vi "Main.vi"() -> ()   [LabVIEW 2024]
uses:
  PIMax3Test01/x64/Debug/PIMax3Test02.dll
panel:
  in  "Accumulations":i64
  out "Accumulations (Get)":i64
  out "Close Camera":string
  out "Intensity Graph 2":u16[][](graph)
  out "Uninit Message":string
  out "model":string
  out "open":string
  out "Init Message":string
  out "Uninit Code":i32
  out "Init Code":i32
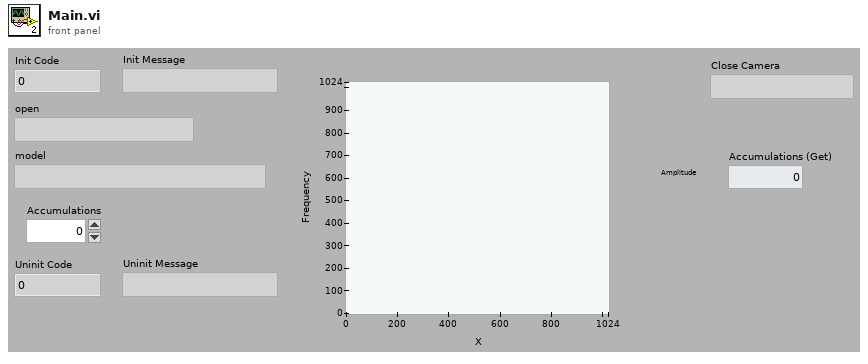
[diagram p1: front panel]
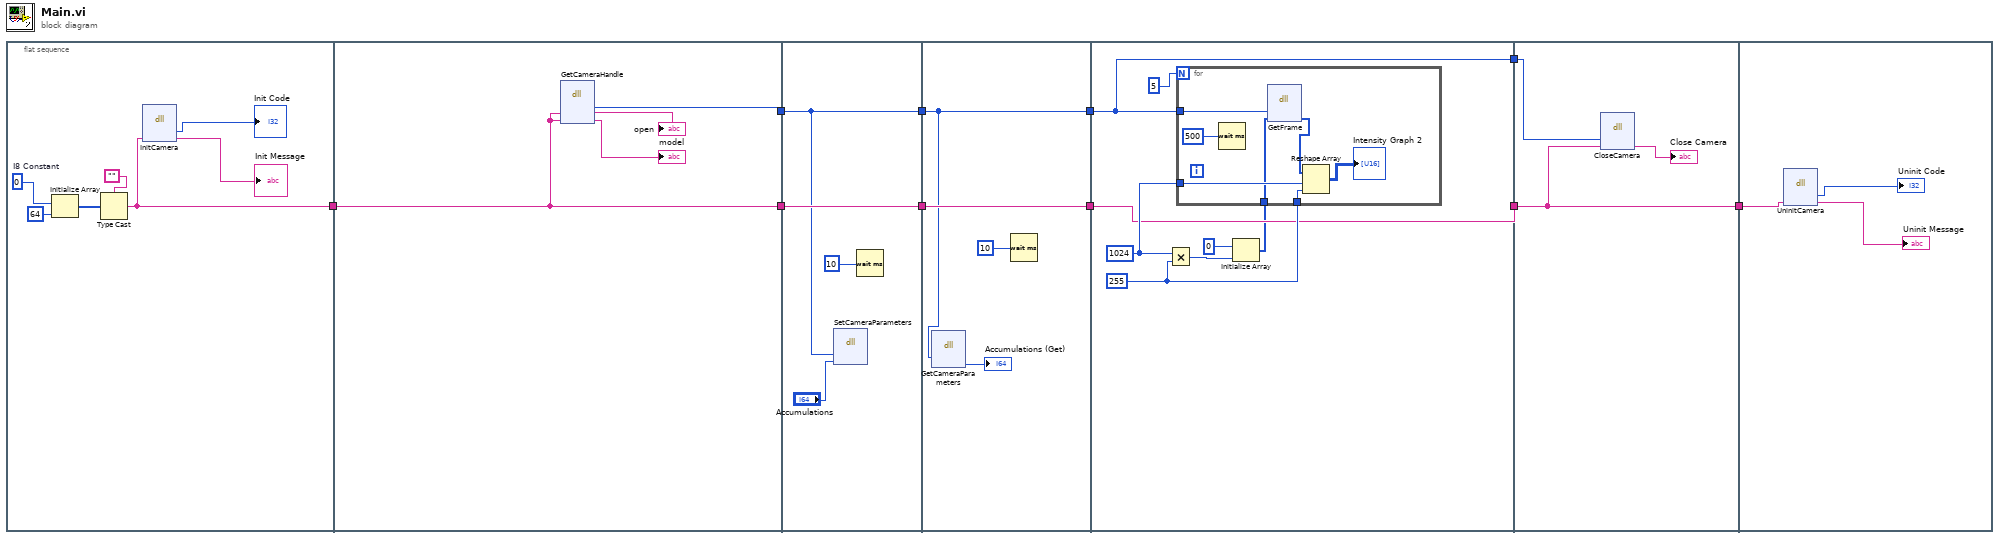
[diagram p0: block diagram]
diagram:
  n1 = flat-sequence {
    tunnel: [w11] -> w10
    tunnel: w10 -> [w21]
    tunnel: [w21] -> w6
    tunnel: [w18] -> w5
    tunnel: w6 -> [w25]
    tunnel: [w25] -> w4
    tunnel: w5 -> [w24]
    tunnel: [w24] -> w2
    tunnel: w4 -> [w29]
    tunnel: [w29] -> w3
    tunnel: w2 -> [w27]
    tunnel: [w27] -> w1
    tunnel: w3 -> [w33]
    tunnel: [w33] -> w9
    tunnel: w1 -> [w30]
    tunnel: [w30] -> w7
    tunnel: w9 -> [w47]
    tunnel: [w47] -> w8
    tunnel: w7 -> [w45]
    tunnel: w8 -> [w49]
    frame #0 {
      w16 = i8 0  # I8 Constant
      n2 = Initialize Array(w16, 64 ("dimension size")) -> (w15:i8[])
      n3 = Type Cast(type="", x=w15) -> (*(type *) &x=w11:string)
      n4 = dll-call lib="C:/Users/amir0/source/repos/PIMax3Test01/x64/Debug/PIMax3Test02.dll" fn="InitCamera"("Init Message"=w11) -> ("Init Code"=→"Init Code":i32, "Init Message"=→"Init Message":string)  [unwired: 5 in, 2 out]
    }
    frame #1 {
      n5 = dll-call lib="C:/Users/amir0/source/repos/PIMax3Test01/x64/Debug/PIMax3Test02.dll" fn="GetCameraHandle"("Open Camera"=w21, "Sensor Name"=w21) -> ("Camera Handle"=w18:u64, "Open Camera"=→"open":string, "Sensor Name"=→"model":string)  [unwired: 5 in, 2 out]
    }
    frame #2 {
      n6 = dll-call lib="C:/Users/amir0/source/repos/PIMax3Test01/x64/Debug/PIMax3Test02.dll" fn="SetCameraParameters"("Camera Handle"=w24, "Accumulations"="Accumulations") -> ()  [unwired: 6 in, 2 out]
      n7 = Wait (ms)(milliseconds to wait=u32 10) -> ()  [unwired: 1 out]
    }
    frame #3 {
      n8 = dll-call lib="C:/Users/amir0/source/repos/PIMax3Test01/x64/Debug/PIMax3Test02.dll" fn="GetCameraParameters"("Camera Handle"=w27) -> ("Accumulations"=→"Accumulations (Get)":i64)  [unwired: 6 in, 2 out]
      n9 = Wait (ms)(milliseconds to wait=u32 10) -> ()  [unwired: 1 out]
    }
    frame #4 {
      w36 = 255
      w35 = 1024
      n10 = Multiply(x=w35, y=w36) -> (x*y=w37:i32)
      n11 = Initialize Array(u16 0, w37) -> (w32:u16[])
      n12 = for {
        N: 5 -> [_]
        tunnel: w36 -> [w44]
        tunnel: w35 -> [w43]
        tunnel: w30 -> [w42]
        tunnel: w32 -> [w41]
        n13 = Wait (ms)(milliseconds to wait=u32 500) -> ()  [unwired: 1 out]
        n14 = dll-call lib="C:/Users/amir0/source/repos/PIMax3Test01/x64/Debug/PIMax3Test02.dll" fn="GetFrame"("Camera Handle"=w42, "Image"=w41) -> ("Image"=w40:u16[])  [unwired: 5 in, 2 out]
        n15 = Reshape Array(w40, w43, w44) -> (→"Intensity Graph 2":u16[][])
      }
    }
    frame #5 {
      n16 = dll-call lib="C:/Users/amir0/source/repos/PIMax3Test01/x64/Debug/PIMax3Test02.dll" fn="CloseCamera"("Camera Handle"=w45, "Close Camera"=w47) -> ("Close Camera"=→"Close Camera":string)  [unwired: 5 in, 2 out]
    }
    frame #6 {
      n17 = dll-call lib="C:/Users/amir0/source/repos/PIMax3Test01/x64/Debug/PIMax3Test02.dll" fn="UninitCamera"("Uninit Message"=w49) -> ("Uninit Code"=→"Uninit Code":i32, "Uninit Message"=→"Uninit Message":string)  [unwired: 5 in, 2 out]
    }
  }
